vi "STOP_Motor.vi"(6 "error in (no error)":errorcluster, 9 "TCP Network Connection in":refnum<k5>) -> (0 "error out":errorcluster, 3 "TCP Network Connection out":refnum<k5>)   [LabVIEW 2019]
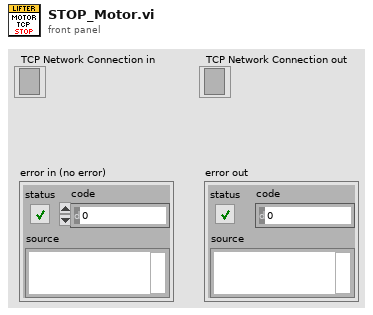
[diagram p1: front panel]
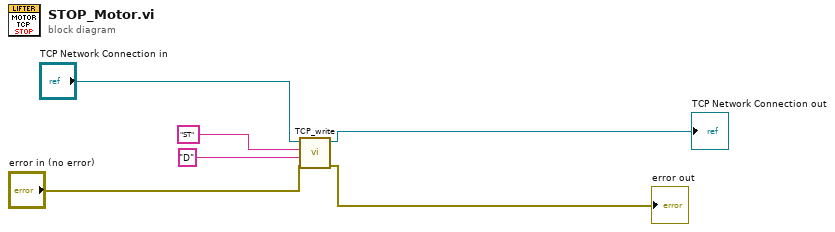
[diagram p0: block diagram]
diagram:
  n1 = call "TCP_write.vi"("error in"="error in (no error)", "Parameter 2"="D", "Parameter 1"="ST" ("string"), "connection ID"="TCP Network Connection in") -> ("error out"=→"error out":errorcluster, "TCP Network Connection out"=→"TCP Network Connection out":refnum<k5>)  [unwired: 5 in, 1 out]
